vi "TransformAngle.vi"(1 "Angle":dbl, 2 "XY Vector":dbl[](array[numeric])) -> (0 "Result Vector":dbl[](array[numeric]))   [LabVIEW 2015]
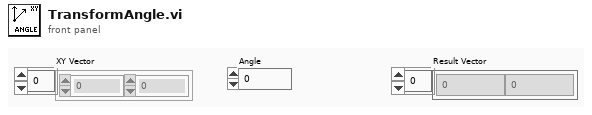
[diagram p1: front panel]
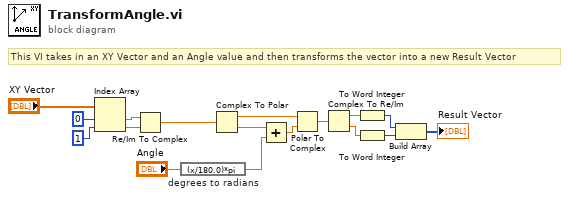
[diagram p0: block diagram]
diagram:
  # "This VI takes in an XY Vector and an Angle value and then transforms the vector into a new Result Vector"
  n1 = Index Array(array="XY Vector", index #1=0 ("index"), index #2=1) -> (element #1=w6:dbl, element #2=w7:dbl)
  n2 = Re/Im To Complex(1:w7, 2:w6) -> (0:w14:cdb)
  n3 = expression code="(x/180.0)*pi" "degrees to radians"("Angle") -> (w8:dbl)
  n4 = Complex To Polar(r * e^(i*theta)=w14) -> (r=w12:dbl, theta=w13:dbl)
  n5 = Add(x=w13, y=w8) -> (x+y=w11:dbl)
  n6 = Polar To Complex(1:w11, 2:w12) -> (0:w10:cdb)
  n7 = Complex To Re/Im(x + iy=w10) -> (x=w4:dbl, y=w5:dbl)
  n8 = To Word Integer(number=w4) -> (16bit integer=w3:i16)
  n9 = To Word Integer(number=w5) -> (16bit integer=w2:i16)
  n10 = Build Array(w3, w2) -> (→"Result Vector":i16[])
